vi "Get Database.vi"(8 "error in (no error)":errorcluster, 11 "Table in":refnum<class "Basic Table.lvclass">) -> (0 "error out":errorcluster, 2 "Database Out":refnum<class "Database Interface.lvclass">, 3 "Table out":refnum<class "Basic Table.lvclass">)   [LabVIEW 2020, in "Table.lvlib" / "Basic Table.lvclass"]
uses:
  Basic Table.lvclass
  Database Libraries/Database Interfaces/Database Interface Class/Database Interface.lvclass
  Basic Table.lvclass/Basic Table.ctl
  Table Configuration Interface/Table Configuration Interface.lvclass
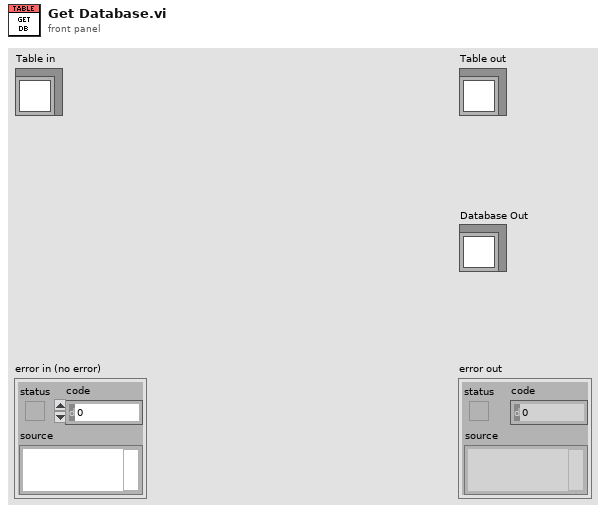
[diagram p1: front panel]
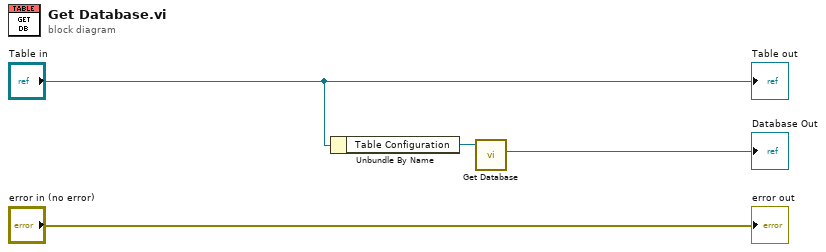
[diagram p0: block diagram]
diagram:
  n1 = Unbundle By Name("Table in") -> ("Table Configuration"=w2:refnum<class "Table Configuration Interface.lvclass">)
  n2 = call-dynamic "Get Database.vi"("Table Configuration Interface in"=w2) -> ("Database"=→"Database Out":refnum<class "Database Interface.lvclass">)  [unwired: 8 in, 2 out]
  "error out" <- "error in (no error)"
  "Table out" <- "Table in"
